vi "fit function selector - new.vi"(5 "fit using":T3=enum."varshni", 7 "fit action":T2=enum."calc", 9 "y":dbl[](array[numeric]), 10 "x":dbl[](array[numeric]), 11 "fit parameters":dbl[](array[numeric])) -> (0 "vi reference":T1, 1 "y out":dbl[](array[numeric]), 2 "x out":dbl[](array[numeric]), 3 "fit params out":dbl[](array[numeric]), 4 "fit function name":string="varshni fit function.vi")   [LabVIEW 2015]
uses:
  fit function selector control.ctl
  array -- fit control .ctl
  <vilib>/gmath/NumericalOptimization/LM model function reference.ctl
  <vilib>/gmath/NI_Gmath.lvlib
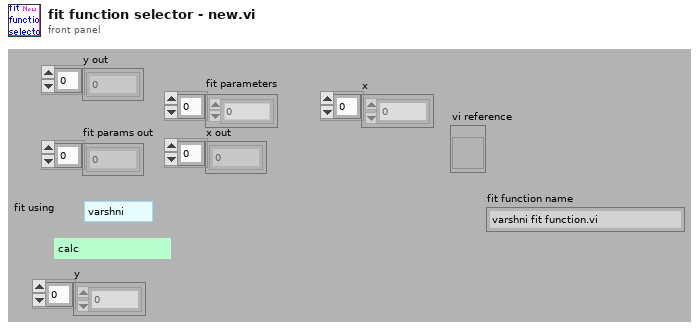
[diagram p1: front panel]
types:
  T1 = typedef "NI_Gmath.lvlib/LM model function reference.ctl" = refnum<vi>
  T2 = typedef "array -- fit control .ctl" = enum16{"fit", "calc", "check", "init"}
  T3 = typedef "fit function selector control.ctl" = enum16{"linear", "varshni", "varshni5", "LogMinusT", "hyperbola", "einstein", "sine", "sine2theta", "cos2theta"}
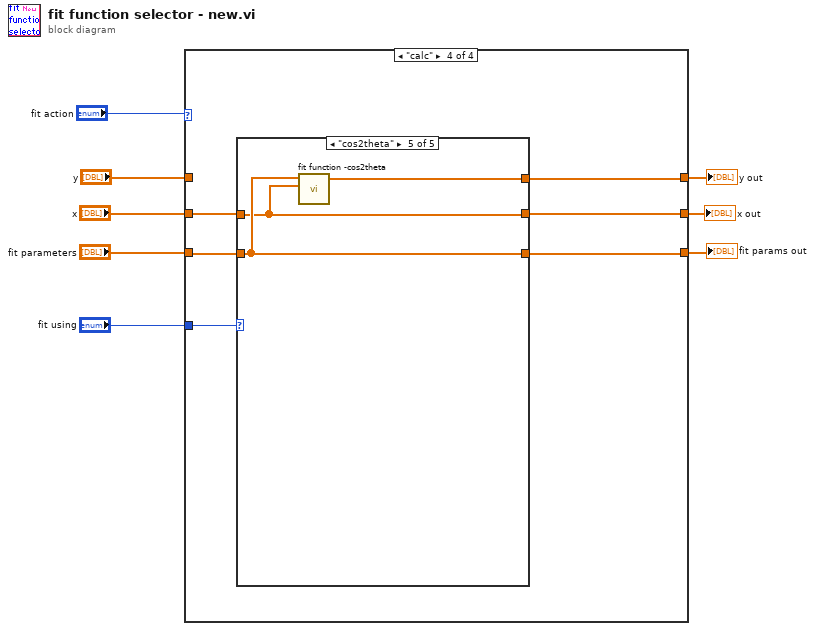
[diagram p0: block diagram]
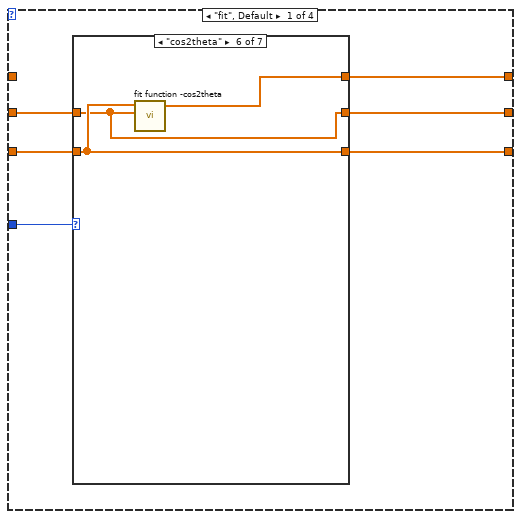
[diagram p2: hidden frame]
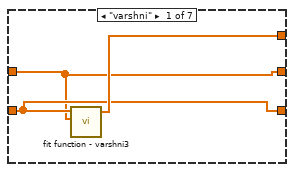
[diagram p3: hidden frame]
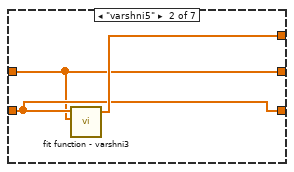
[diagram p4: hidden frame]
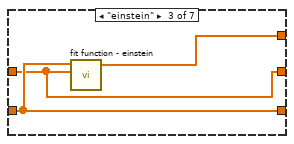
[diagram p5: hidden frame]
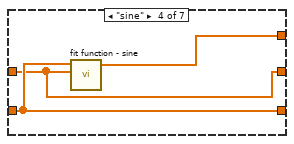
[diagram p6: hidden frame]
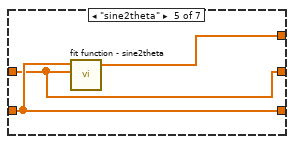
[diagram p7: hidden frame]
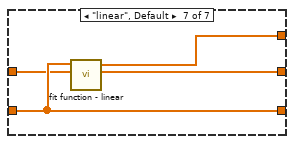
[diagram p8: hidden frame]
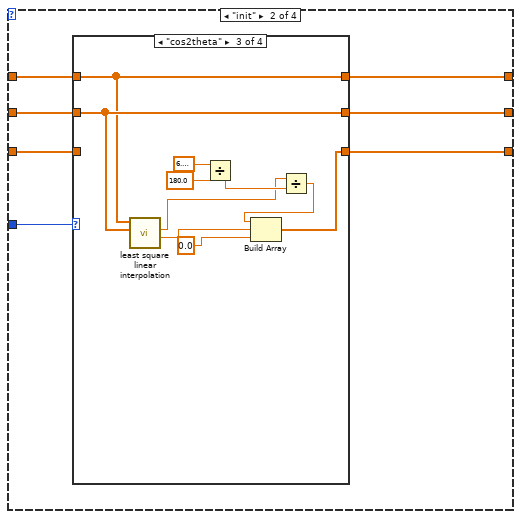
[diagram p9: hidden frame]
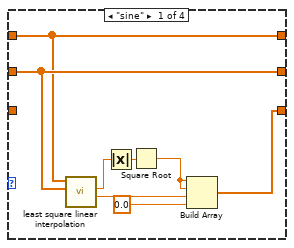
[diagram p10: hidden frame]
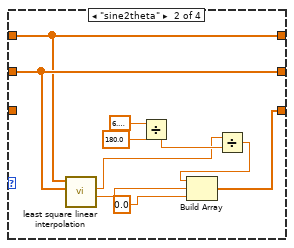
[diagram p11: hidden frame]
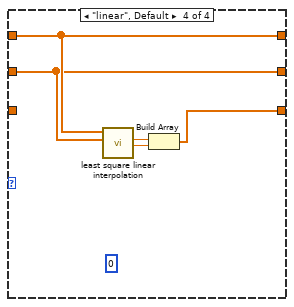
[diagram p12: hidden frame]
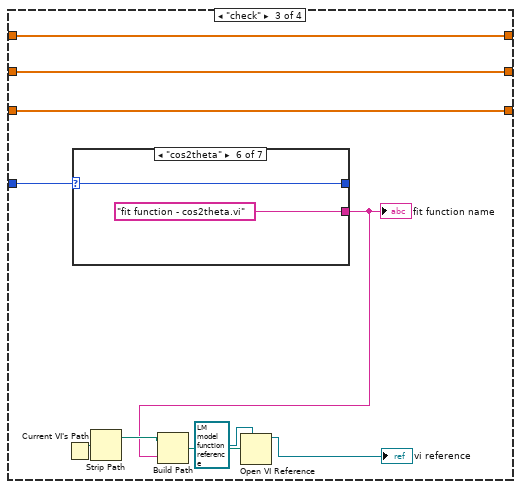
[diagram p13: hidden frame]
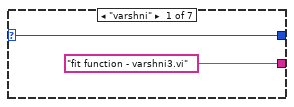
[diagram p14: hidden frame]
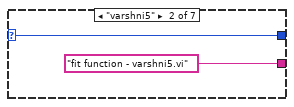
[diagram p15: hidden frame]
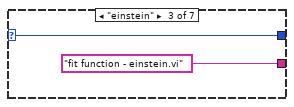
[diagram p16: hidden frame]
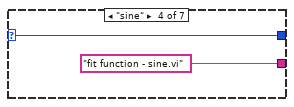
[diagram p17: hidden frame]
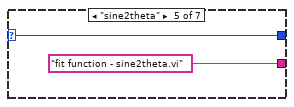
[diagram p18: hidden frame]
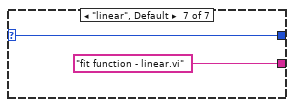
[diagram p19: hidden frame]
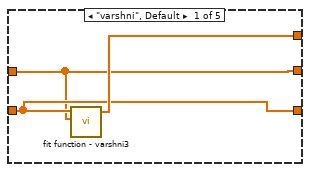
[diagram p20: hidden frame]
diagram:
  n1 = case shown="\"calc\"" "fit action" {
    tunnel: "x" -> [w14 w42 w78 w104]
    tunnel: [w13 w41 w77 w100] -> w7
    tunnel: [w12 w40 w76 w101] -> w6
    tunnel: "fit using" -> [w11 w39 w85 w105]
    tunnel: "fit parameters" -> [w10 w38 w76 w103]
    tunnel: [w9 w37 w78 w102] -> w3
    tunnel: "y" -> [_ w36 w77 _]
    frame "fit", Default {
      n2 = case shown="\"cos2theta\"" w11 {
        tunnel: w10 -> [w16 w19 w22 w25 w28 w31 w34]
        tunnel: w14 -> [w15 w18 w21 w24 w27 w30 w33]
        tunnel: [w17 w20 w23 w26 w29 w32 w35] -> w13
        tunnel: [w16 w19 w22 w25 w28 w31 w34] -> w12
        tunnel: [w15 w18 w21 w24 w27 w30 w33] -> w9
        frame "varshni" {
          n3 = call "fit function - varshni3.vi"("X"=w15, "a"=w16) -> ("f(X,a)"=w17:dbl[])  [unwired: 2 in, 2 out]
        }
        frame "varshni5" {
          n4 = call "fit function - varshni3.vi"("X"=w18, "a"=w19) -> ("f(X,a)"=w20:dbl[])  [unwired: 2 in, 2 out]
        }
        frame "einstein" {
          n5 = call "fit function - einstein.vi"("X"=w21, "a"=w22) -> ("f(X,a)"=w23:dbl[])  [unwired: 2 in, 2 out]
        }
        frame "sine" {
          n6 = call "fit function - sine.vi"("X"=w24, "a"=w25) -> ("f(X,a)"=w26:dbl[])  [unwired: 2 in, 2 out]
        }
        frame "sine2theta" {
          n7 = call "fit function - sine2theta.vi"("X"=w27, "a"=w28) -> ("f(X,a)"=w29:dbl[])  [unwired: 2 in, 2 out]
        }
        frame "cos2theta" {
          n8 = call "fit function -cos2theta.vi"("X"=w30, "a"=w31) -> ("f(X,a)"=w32:dbl[])  [unwired: 2 in, 2 out]
        }
        frame "linear", Default {
          n9 = call "fit function - linear.vi"("X"=w33, "a"=w34) -> ("f(X,a)"=w35:dbl[])  [unwired: 2 in, 2 out]
        }
      }
    }
    frame "init" {
      n10 = case shown="\"cos2theta\"" w39 {
        tunnel: w38 -> [_ _ _ _]
        tunnel: w42 -> [w50 w60 w70 w72]
        tunnel: [w49 w59 w69 w73] -> w41
        tunnel: [w48 w58 w68 w71] -> w40
        tunnel: [w50 w60 w70 w72] -> w37
        tunnel: w36 -> [w49 w59 w69 w73]
        frame "sine" {
          n11 = call "least square linear interpolation.vi"("X"=w50, "Y"=w49) -> ("intercept"=w44:dbl, "slope"=w47:dbl)  [unwired: 8 in]
          n12 = Absolute Value(x=w47) -> (abs(x)=w46:dbl)
          n13 = Square Root(x=w46) -> (sqrt(x)=w45:dbl)
          n14 = Build Array(w45, w45, w44, 0.0 ("element")) -> (w48:dbl[])
        }
        frame "sine2theta" {
          n15 = call "least square linear interpolation.vi"("X"=w60, "Y"=w59) -> ("intercept"=w57:dbl, "slope"=w51:dbl)  [unwired: 8 in]
          n16 = Divide(x=6.283185307179586, y=180.0) -> (x/y=w53:dbl)
          n17 = Divide(x=w51, y=w53) -> (x/y=w52:dbl)
          n18 = Build Array(w52, w57, 0.0 ("element")) -> (w58:dbl[])
        }
        frame "cos2theta" {
          n19 = call "least square linear interpolation.vi"("X"=w70, "Y"=w69) -> ("intercept"=w67:dbl, "slope"=w61:dbl)  [unwired: 8 in]
          n20 = Divide(x=6.283185307179586, y=180.0) -> (x/y=w63:dbl)
          n21 = Divide(x=w61, y=w63) -> (x/y=w62:dbl)
          n22 = Build Array(w62, w67, 0.0 ("element")) -> (w68:dbl[])
        }
        frame "linear", Default {
          (unwired) 0
          n23 = call "least square linear interpolation.vi"("X"=w72, "Y"=w73) -> ("intercept"=w74:dbl, "slope"=w75:dbl)  [unwired: 8 in]
          n24 = Build Array(w75, w74) -> (w71:dbl[])
        }
      }
    }
    frame "check" {
      n25 = Current VI's Path() -> (path=w82:path)
      n26 = case shown="\"cos2theta\"" w85 {
        selector: w85 -> [w87 w89 w91 w93 w95 w97 w99]
        tunnel: ["fit function - varshni3.vi" ("f(x,a) VI name Complex") "fit function - varshni5.vi" ("f(x,a) VI name Complex") "fit function - einstein.vi" ("f(x,a) VI name Complex") "fit function - sine.vi" ("f(x,a) VI name Complex") "fit function - sine2theta.vi" ("f(x,a) VI name Complex") "fit function - cos2theta.vi" ("f(x,a) VI name Complex") "fit function - linear.vi" ("f(x,a) VI name Complex")] -> w80
        tunnel: [w87 w89 w91 w93 w95 w97 w99] -> _
        frame "varshni" {
        }
        frame "varshni5" {
        }
        frame "einstein" {
        }
        frame "sine" {
        }
        frame "sine2theta" {
        }
        frame "cos2theta" {
        }
        frame "linear", Default {
        }
      }
      "fit function name" <- w80
      n27 = Strip Path(path=w82) -> (stripped path=w81:path)  [unwired: 1 out]
      n28 = Build Path(base path=w81, name or relative path=w80) -> (appended path=w84:path)
      n29 = Open VI Reference(type specifier VI Refnum (for type only)=T1 refnum ("f(x,a)"), vi path=w84) -> (vi reference=→"vi reference":T1)  [unwired: 1 in, 4 out]
    }
    frame "calc" {
      n30 = case shown="\"cos2theta\"" w105 {
        tunnel: w103 -> [w107 w110 w113 w116 w119]
        tunnel: w104 -> [w106 w109 w112 w115 w118]
        tunnel: [w108 w111 w114 w117 w120] -> w100
        tunnel: [w107 w110 w113 w116 w119] -> w101
        tunnel: [w106 w109 w112 w115 w118] -> w102
        frame "varshni", Default {
          n31 = call "fit function - varshni3.vi"("X"=w106, "a"=w107) -> ("f(X,a)"=w108:dbl[])  [unwired: 2 in, 2 out]
        }
        frame "einstein" {
          n32 = call "fit function - einstein.vi"("X"=w109, "a"=w110) -> ("f(X,a)"=w111:dbl[])  [unwired: 2 in, 2 out]
        }
        frame "sine" {
          n33 = call "fit function - sine.vi"("X"=w112, "a"=w113) -> ("f(X,a)"=w114:dbl[])  [unwired: 2 in, 2 out]
        }
        frame "sine2theta" {
          n34 = call "fit function - sine2theta.vi"("X"=w115, "a"=w116) -> ("f(X,a)"=w117:dbl[])  [unwired: 2 in, 2 out]
        }
        frame "cos2theta" {
          n35 = call "fit function -cos2theta.vi"("X"=w118, "a"=w119) -> ("f(X,a)"=w120:dbl[])  [unwired: 2 in, 2 out]
        }
      }
    }
  }
  "y out" <- w7
  "fit params out" <- w6
  "x out" <- w3
